vi "waitOnTask.vi"(0 "HGF_ThreadPool_Reference":refnum<class "HGF_Reference.lvclass">, 3 "timeout in ms (-1)":i32=-1, 5 "error in (no error)":errorcluster) -> (14 "dup HGF_ThreadPool_Reference":refnum<class "HGF_Reference.lvclass">, 16 "HGF_Task":refnum<class "HGF_ThreadTask.lvclass">, 17 "timed out?":bool, 19 "error out":errorcluster)   [LabVIEW 2014, in "HGF_BaseClasses.lvlib" / "HGF_ThreadPool.lvclass"]
doc: "Wait on completed HGF_Task."
uses:
  HGF_ThreadPool.lvclass
  HGF_Reference/HGF_Reference.lvclass
  HGF_ThreadTask/HGF_ThreadTask.lvclass
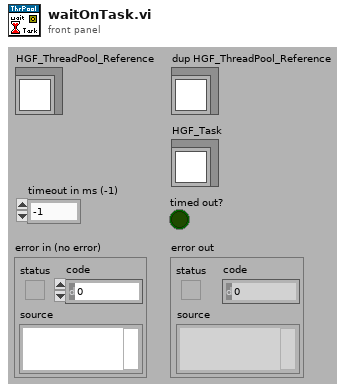
[diagram p1: front panel]
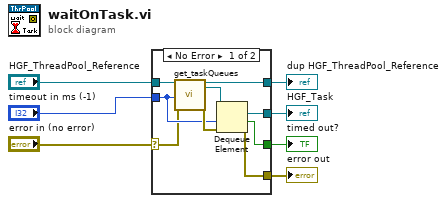
[diagram p0: block diagram]
diagram:
  n1 = case shown="No Error" "error in (no error)" {
    selector: "error in (no error)" -> [w11 w18]
    tunnel: [w10 w18] -> w6
    tunnel: [w13 w17] -> w3
    tunnel: "HGF_ThreadPool_Reference" -> [w14 w17]
    tunnel: "timeout in ms (-1)" -> [w12 _]
    tunnel: [w9 _] -> w2
    tunnel: [w8 _] -> w1
    frame No Error {
      n2 = call "get_taskQueues.vi"("HGF_ThreadPool_Reference"=w14, "timeout in ms (-1)"=w12, "error in (no error)"=w11) -> ("dup HGF_ThreadPool_Reference"=w13:refnum<class "HGF_Reference.lvclass">, "taskQueue out"=w15:refnum<queue>, "error out"=w16:errorcluster)  [unwired: 14 out]
      n3 = Dequeue Element(queue=w15, timeout in ms (-1)=w12, error in (no error)=w16) -> (element=w9:refnum<class "HGF_ThreadTask.lvclass">, timed out?=w8:bool, error out=w10:errorcluster)  [unwired: 1 out]
    }
    frame Error {
    }
  }
  "error out" <- w6
  "dup HGF_ThreadPool_Reference" <- w3
  "HGF_Task" <- w2
  "timed out?" <- w1
